vi "Drive Direction.vi"(6 "Wheel DevRef":T1={"DeviceStatus"={"status"=FALSE, "code"=0, "source"=""}, "Type"=enum."PWM", "PWM"={"PWM Channel"=enum."Invalid", "DeadBand"={"Name"="", "maxPositivePwm"=0, "minPositivePwm"=0, "centerPwm"=0, "maxNegativePwm"=0, "minNegativePwm"=0, "angularRange"=0}}, "CAN"={"Device Number"=0, "SetOutput VI Ref"=variant(refnum<vi> refnum), "GetOutput VI Ref"=variant(refnum<vi> refnum), "Enable VI Ref"=variant(refnum<vi> refnum), "Disable VI Ref"=variant(refnum<vi> refnum), "Data"=variant}, "Invert"=FALSE}, 7 "Swerve DevRef":T1={"DeviceStatus"={"status"=FALSE, "code"=0, "source"=""}, "Type"=enum."PWM", "PWM"={"PWM Channel"=enum."PWM 1", "DeadBand"={"Name"="", "maxPositivePwm"=0, "minPositivePwm"=0, "centerPwm"=0, "maxNegativePwm"=0, "minNegativePwm"=0, "angularRange"=0}}, "CAN"={"Device Number"=0, "SetOutput VI Ref"=variant(enum8{"Percent VBus", "Current", "Speed", "Position", "Voltage"} enum."Percent VBus"), "GetOutput VI Ref"=variant(refnum<k1> refnum), "Enable VI Ref"=variant(dbl 12.0), "Disable VI Ref"=variant(enum8{"Percent VBus", "Speed", "Position", "Slave", "Unchanged / Invalid", "Voltage Compensation", "Current", "Motion Profile"} enum."Percent VBus"), "Data"=variant}, "Invert"=FALSE}, 8 "error in":errorcluster, 9 "Wheel Power":dbl format="%#_13g", 10 "Desired direction (radians)":dbl=6.283185307179586 format="%#_13g") -> (0 "error out":errorcluster, 1 "Setpoint":dbl, 2 "Wheel Speed":dbl, 3 "Swerve Speed":dbl)   [LabVIEW 2016]
uses:
  <vilib>/Rock Robotics/WPI/MotorControl/WPI_MotorControlDeviceRef.ctl
  <vilib>/Rock Robotics/WPI/MotorControl/WPI_MotorControlType.ctl
  <vilib>/Rock Robotics/SystemInterfaces/DIO/FPGA_DIOPWMChannel.ctl
  <vilib>/Rock Robotics/WPI/PWM/WPI_PWMDeadband.ctl
  Main/Robot Global Data.vi
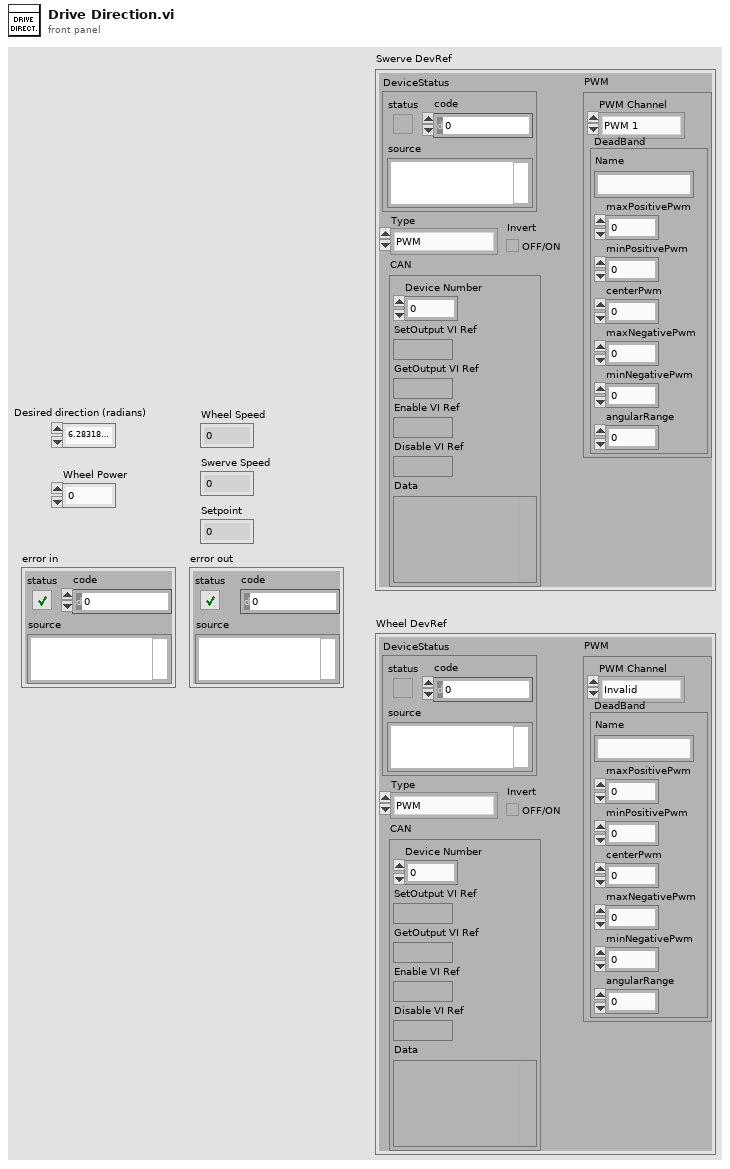
[diagram p1: front panel]
types:
  T1 = typedef "WPI_MotorControlDeviceRef.ctl" = cluster{"DeviceStatus":errorcluster, "Type":T2, "PWM":cluster{"PWM Channel":T3, "DeadBand":T4}, "CAN":cluster{"Device Number":u8, "SetOutput VI Ref":variant, "GetOutput VI Ref":variant, "Enable VI Ref":variant, "Disable VI Ref":variant, "Data":variant}, "Invert":bool}
  T2 = typedef "WPI_MotorControlType.ctl" = enum16{"PWM", "CAN"}
  T3 = typedef "FPGA_DIOPWMChannel.ctl" = enum8{"PWM 0", "PWM 1", "PWM 2", "PWM 3", "PWM 4", "PWM 5", "PWM 6", "PWM 7", "PWM 8", "PWM 9", "PWM MXP 0", "PWM MXP 1", "PWM MXP 2", "PWM MXP 3", "PWM MXP 4", "PWM MXP 5", "PWM MXP 6", "PWM MXP 7", "PWM MXP 8", "PWM MXP 9", "Invalid"}
  T4 = typedef "WPI_PWMDeadband.ctl" = cluster{"Name":string, "maxPositivePwm":i32, "minPositivePwm":i32, "centerPwm":i32, "maxNegativePwm":i32, "minNegativePwm":i32, "angularRange":u16}
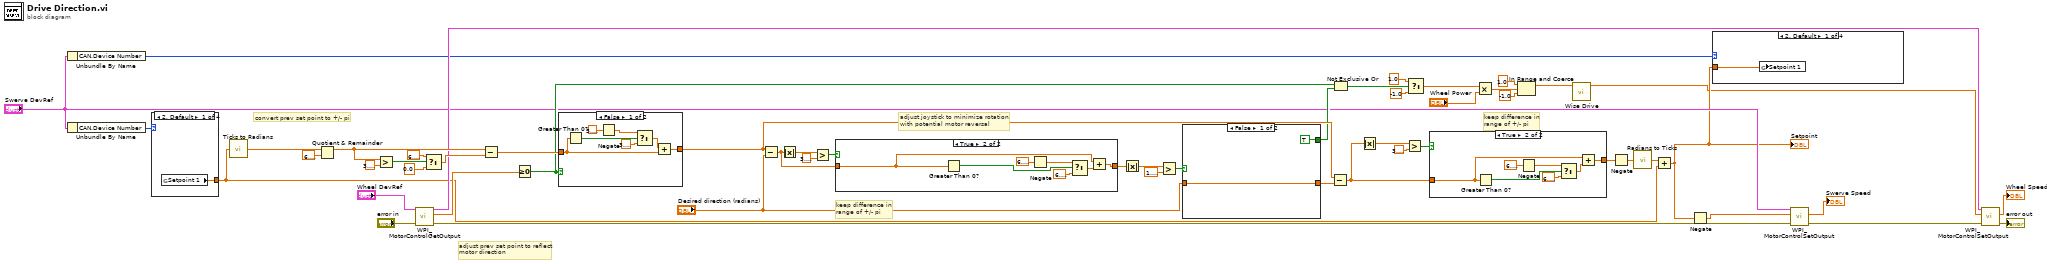
[diagram p0: block diagram]
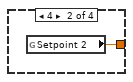
[diagram p2: hidden frame]
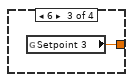
[diagram p3: hidden frame]
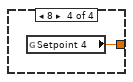
[diagram p4: hidden frame]
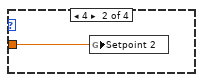
[diagram p5: hidden frame]
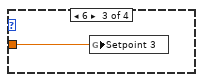
[diagram p6: hidden frame]
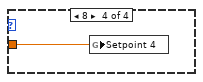
[diagram p7: hidden frame]
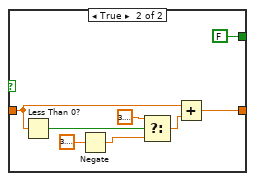
[diagram p9: hidden frame]
diagram:
  # "keep difference in\nrange of +/- pi"
  # "adjust joystick to minimize rotation\nwith potential motor reversal"
  # "keep difference in\nrange of +/- pi"
  # "adjust prev set point to reflect\nmotor direction"
  # "convert prev set point to +/- pi"
  n1 = Unbundle By Name("Swerve DevRef") -> ("CAN.Device Number"=w13:u8)
  n2 = Unbundle By Name("Swerve DevRef") -> ("CAN.Device Number"=w12:u8)
  n3 = case shown="2, Default" w12 {
    tunnel: [w55 w56 w57 w58] -> w11
    frame 2, Default {
      n4 = global read "Robot Global Data.vi" "Setpoint 1"() -> (w55:dbl)
    }
    frame 4 {
      n5 = global read "Robot Global Data.vi" "Setpoint 2"() -> (w56:dbl)
    }
    frame 6 {
      n6 = global read "Robot Global Data.vi" "Setpoint 3"() -> (w57:dbl)
    }
    frame 8 {
      n7 = global read "Robot Global Data.vi" "Setpoint 4"() -> (w58:dbl)
    }
  }
  n8 = call "Ticks to Radians.vi"("Ticks"=w11) -> ("Radians"=w42:dbl)
  n9 = Quotient & Remainder(x=w42, y=6.283185307179586) -> (x-y*floor(x/y)=w48:dbl)  [unwired: 1 out]
  n10 = Greater?(x=w48, y=3.141592653589793) -> (0:w52:bool)
  n11 = call <vilib>:"WPI_MotorControlGetOutput.vi"("error in"="error in", "MotorControlDevRef"="Wheel DevRef") -> ("error out"=w9:errorcluster, "Output"=w35:dbl, "MotorControlDevRef"=w34:T1)  [unwired: 7 in]
  n12 = Select(t=6.283185307179586, s=w52, f=0.0) -> (s? t:f=w49:dbl)
  n13 = Subtract(x=w48, y=w49) -> (x-y=w44:dbl)
  n14 = Greater Or Equal To 0?(x=w35) -> (x >= 0?=w43:bool)
  n15 = case shown="False" w43 {
    tunnel: w44 -> [w60 w66]
    tunnel: [w59 w66] -> w29
    frame False {
      n16 = Greater Than 0?(x=w60) -> (x > 0?=w65:bool)
      n17 = Negate(x=3.141592653589793) -> (-x=w64:dbl)
      n18 = Select(t=w64, s=w65, f=3.141592653589793) -> (s? t:f=w61:dbl)
      n19 = Add(x=w61, y=w60) -> (x+y=w59:dbl)
    }
    frame True {
    }
  }
  n20 = Subtract(x=w29, y="Desired direction (radians)") -> (x-y=w31:dbl)
  n21 = Absolute Value(x=w31) -> (abs(x)=w45:dbl)
  n22 = Greater?(x=w45, y=3.141592653589793) -> (0:w47:bool)
  n23 = case shown="True" w47 {
    tunnel: w31 -> [w67 w69]
    tunnel: [w67 w68] -> w30
    frame False {
    }
    frame True {
      n24 = Greater Than 0?(x=w69) -> (x > 0?=w74:bool)
      n25 = Negate(x=6.283185307179586) -> (-x=w71:dbl)
      n26 = Select(t=w71, s=w74, f=6.283185307179586) -> (s? t:f=w70:dbl)
      n27 = Add(x=w69, y=w70) -> (x+y=w68:dbl)
    }
  }
  n28 = Absolute Value(x=w30) -> (abs(x)=w4:dbl)
  n29 = Greater?(x=w4, y=1.5707963267948966) -> (0:w3:bool)
  n30 = case shown="False" w3 {
    tunnel: "Desired direction (radians)" -> [w76 w79]
    tunnel: [w76 w78] -> w28
    tunnel: [TRUE FALSE] -> w27
    frame False {
    }
    frame True {
      n31 = Less Than 0?(x=w79) -> (x < 0?=w84:bool)
      n32 = Negate(x=3.141592653589793) -> (-x=w81:dbl)
      n33 = Select(t=3.141592653589793, s=w84, f=w81) -> (s? t:f=w80:dbl)
      n34 = Add(x=w79, y=w80) -> (x+y=w78:dbl)
    }
  }
  n35 = Subtract(x=w29, y=w28) -> (x-y=w23:dbl)
  n36 = Not Exclusive Or(1:w27, 2:w43) -> (0:w41:bool)
  n37 = Absolute Value(x=w23) -> (abs(x)=w26:dbl)
  n38 = Greater?(x=w26, y=3.141592653589793) -> (0:w25:bool)
  n39 = Select(t=1.0, s=w41, f=-1.0 ("t")) -> (s? t:f=w38:dbl)
  n40 = case shown="True" w25 {
    tunnel: w23 -> [w85 w87]
    tunnel: [w85 w86] -> w22
    frame False {
    }
    frame True {
      n41 = Greater Than 0?(x=w87) -> (x > 0?=w92:bool)
      n42 = Negate(x=6.283185307179586) -> (-x=w90:dbl)
      n43 = Select(t=w90, s=w92, f=6.283185307179586) -> (s? t:f=w89:dbl)
      n44 = Add(x=w87, y=w89) -> (x+y=w86:dbl)
    }
  }
  n45 = Multiply(x=w38, y="Wheel Power") -> (x*y=w16:dbl)
  n46 = In Range and Coerce(upper limit=1.0, x=w16, lower limit=-1.0) -> (coerced(x)=w2:dbl)  [unwired: 1 out]
  n47 = call "Wise Drive.vi"("Joystick Control"=w2) -> ("Throttle"=w1:dbl)  [unwired: 9 in, 1 out]
  n48 = Negate(x=w22) -> (-x=w17:dbl)
  n49 = call "Radians to Ticks.vi"("Radians"=w17) -> ("Ticks"=w21:dbl)
  n50 = Add(x=w21, y=w11) -> (x+y=w8:dbl)
  "Setpoint" <- w8
  n51 = Negate(x=w8) -> (-x=w7:dbl)
  n52 = case shown="2, Default" w13 {
    tunnel: w8 -> [w93 w94 w95 w96]
    frame 2, Default {
      n53 = global write "Robot Global Data.vi" "Setpoint 1"(w93) -> ()
    }
    frame 4 {
      n54 = global write "Robot Global Data.vi" "Setpoint 2"(w94) -> ()
    }
    frame 6 {
      n55 = global write "Robot Global Data.vi" "Setpoint 3"(w95) -> ()
    }
    frame 8 {
      n56 = global write "Robot Global Data.vi" "Setpoint 4"(w96) -> ()
    }
  }
  n57 = call <vilib>:"WPI_MotorControlSetOutput.vi"("error in (no error)"=w9, "Output"=w7, "MotorControlDevRef"="Swerve DevRef") -> ("error out"=w5:errorcluster, "Motor Output"=→"Swerve Speed":dbl)  [unwired: 6 in, 1 out]
  n58 = call <vilib>:"WPI_MotorControlSetOutput.vi"("error in (no error)"=w5, "Output"=w1, "MotorControlDevRef"=w34) -> ("error out"=→"error out":errorcluster, "Motor Output"=→"Wheel Speed":dbl)  [unwired: 6 in, 1 out]
